vi "Set Joystick Speed.vi"(8 "error in (no error)":errorcluster, 9 "High Speed Inputs":dbl[](array[numeric]), 10 "Low Speed Inputs":dbl[](array[numeric]), 11 "Gantry":refnum<k24>) -> (0 "error out":errorcluster, 3 "Controller Out":refnum<k24>)   [LabVIEW 2021, in "A3200.lvclass"]
uses:
  A3200.lvclass
  C:/Program Files (x86)/Aerotech/A3200/LabVIEW/2010/Bin/Aerotech.A3200.dll
  Program Files (x86)/Aerotech/A3200/LabVIEW/2010/Bin/Aerotech.A3200.dll
  Drivers/Aerotech A3200/Parameters/SetAxisParameterDouble.vi
  Drivers/Aerotech A3200/Aerotech.lvlib
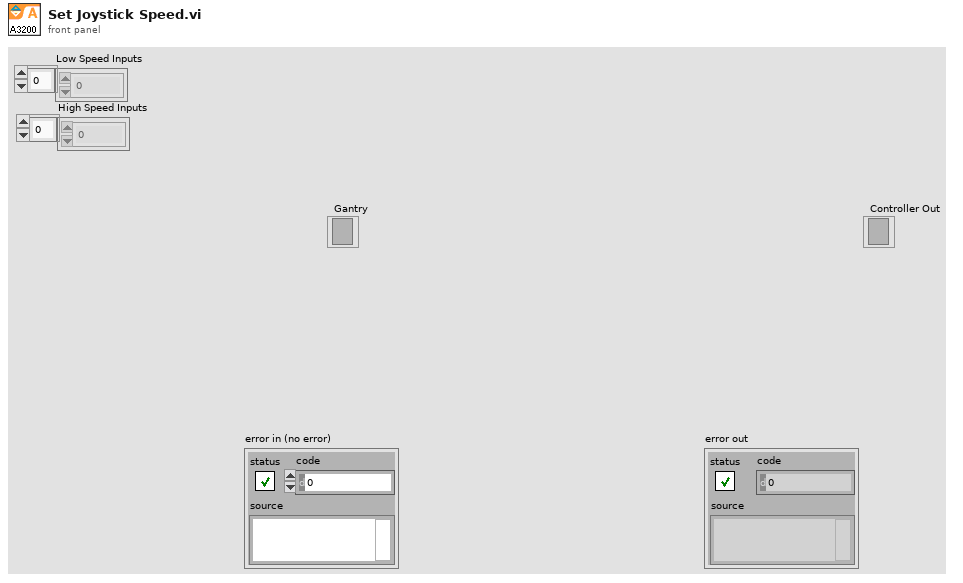
[diagram p1: front panel]
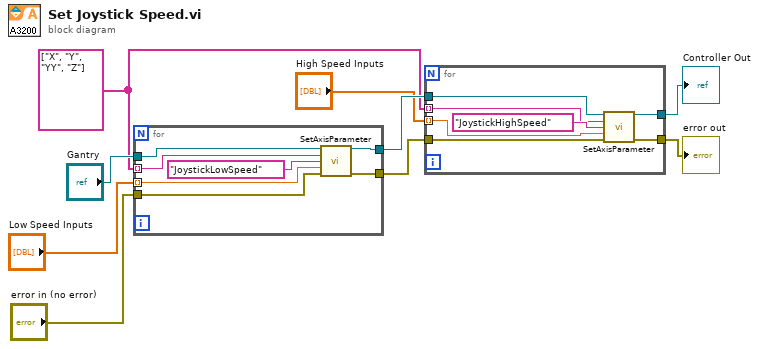
[diagram p0: block diagram]
diagram:
  w4 = string[] ["X", "Y", "YY", "Z"] ("axisName")
  n1 = for {
    tunnel: "Gantry" -> [w16]
    tunnel: "error in (no error)" -> [w14]
    tunnel: [w13] -> w6
    tunnel: [w12] -> w3
    tunnel: w4 -> [w11] mode=indexing
    tunnel: "Low Speed Inputs" -> [w10] mode=indexing
    n2 = call-poly "SetAxisParameter.vi"("Controller In"=w16, "axisName"=w11, "Parameter Name"="JoystickLowSpeed", "value"=w10, "error in (no error)"=w14) -> ("Controller Out"=w13:refnum<k24>, "error out"=w12:errorcluster)  [unwired: 9 in]
  }
  n3 = for {
    tunnel: w6 -> [w23]
    tunnel: w3 -> [w21]
    tunnel: [w20] -> w5
    tunnel: [w19] -> w2
    tunnel: w4 -> [w18] mode=indexing
    tunnel: "High Speed Inputs" -> [w17] mode=indexing
    n4 = call-poly "SetAxisParameter.vi"("Controller In"=w23, "axisName"=w18, "Parameter Name"="JoystickHighSpeed", "value"=w17, "error in (no error)"=w21) -> ("Controller Out"=w20:refnum<k24>, "error out"=w19:errorcluster)  [unwired: 9 in]
  }
  "error out" <- w2
  "Controller Out" <- w5
